vi "ListBox Playground.vi"() -> ()   [LabVIEW 2019]
uses:
  <vilib>/event_ctls.llb/lveventtype.ctl
  <vilib>/event_ctls.llb/eventsource.ctl
  <vilib>/picture/picture.llb/imagedata.ctl
  <vilib>/addons/_JKI Toolkits/Caraya/classes/Test Result/Test Node (Extended).ctl
  <vilib>/addons/_JKI Toolkits/Caraya/classes/Test Result/Test Registration Data.ctl
  <vilib>/Utility/miscctls.llb/LVRowAndColumnUnsignedTypeDef.ctl
  <vilib>/Utility/miscctls.llb/LVRowAndColumnTypeDef.ctl
  <vilib>/addons/_JKI Toolkits/Caraya/classes/Test Result/Test Result.lvclass
panel:
  out "2D Picture 2":picture
  out "image data 2":T1
  out "image data":T1
  out "2D Picture":picture
  out "Ready? 2":bool
  in  "Multicolumn Listbox 2":i32(listbox)
  in  "Patterns":i32(listbox) caption="Patterns (drag-and-drop reorder)"
  out "x = y?":bool
  out "Ctrl":bool
  out "element":string
  out "initialized array":i32[](array[numeric])
  out "Item Names 2":string[][](array[string])
  in  "Multicolumn Listbox":i32(listbox)
  out "Edit Tree Items:Add Item":string
  in  "Tree":string(tree)
  out "Array":string[](array[string])
  out "Item Names":string[](array[string])
  out "Time":u32
  out "Source":T2 items=["LabVIEW UI"=0, "ActiveX"=1, "User Event"=25]
  out "Type":T3=enum."Value Change"
  out "Result":enum16{"Drop Cancel", "Drop Move", "Drop Copy"}(ring)
  out "Drag Ended":bool
  out "Drag Started":bool
  in  "Boolean":bool
  in  "Listbox":i32(listbox)
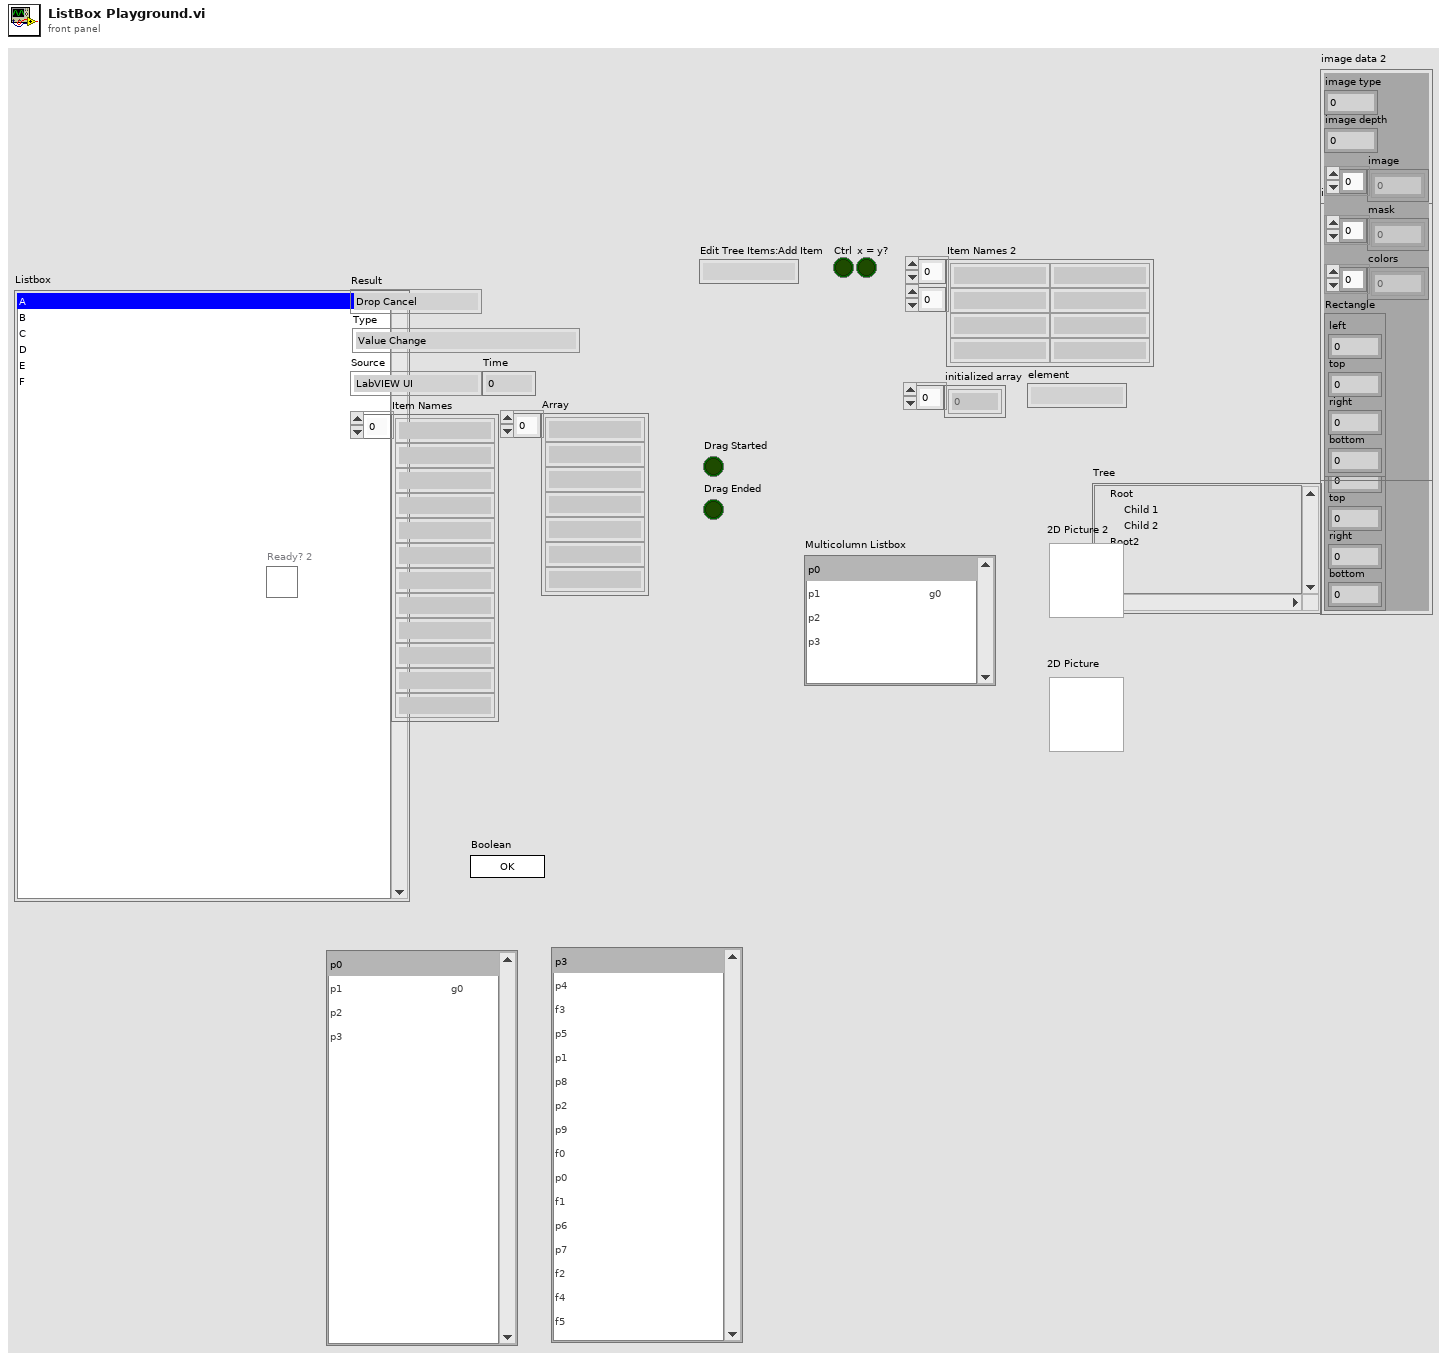
[diagram p1: front panel]
types:
  T1 = typedef "imagedata.ctl" = cluster{"image type":i32, "image depth":i32, "image":u8[], "mask":u8[], "colors":u32[], "Rectangle":cluster{"left":i16, "top":i16, "right":i16, "bottom":i16}}
  T2 = typedef "eventsource.ctl" = u32
  T3 = typedef "lveventtype.ctl" = enum32{"Null", "Timeout", "Annotation Menu Selection", "Annotation Menu Selection?", "App Instance Close", "App Instance Close?", "Autoscale Range Change", "Bookmark Info Change", "Cell Edit", "Cell Edit?", "Cursor Grab", "Cursor Grab?", "Cursor Menu Selection", "Cursor Menu Selection?", "Cursor Move", "Cursor Release", "Data Change", "Direction Change", "Display State Change", "Drag Ended", "Drag Enter", "Drag Leave", "Drag Over", "Drag Source Update", "Drag Starting", "Drag Starting?", "Drop", "Exec State Change", "Key Down", "Key Down?", "Key Repeat", "Key Repeat?", "Key Up", "Listbox Double Click", "Menu Activation?", "Menu Selection (App)", "Menu Selection? (App)", "Menu Selection (User)", "Mouse Down", "Mouse Down?", "Mouse Enter", "Mouse Leave", "Mouse Move", "Mouse Up", "Mouse Wheel", "NI Security User Change (App)", "Pane Size", "Panel Close", "Panel Close?", "Panel Resize", "Plot Attribute Change", "Scale Range Change", "Shortcut Menu Activation?", "Shortcut Menu Selection (App)", "Shortcut Menu Selection? (App)", "Shortcut Menu Selection (User)", "Tree Double Click", "Tree Drag", "Tree Drag?", "Tree Drop", "Tree Drop?", "Tree Item Close", "Tree Item Close?", "Tree Item Open", "Tree Item Open?", "User Event", "Value Change"}
  T4 = cluster{"left":i16, "top":i16, "right":i16, "bottom":i16}
  T5 = typedef "LVRowAndColumnTypeDef.ctl" = cluster{"Row":i32, "Column":i32}
  T6 = typedef "LVRowAndColumnUnsignedTypeDef.ctl" = cluster{"Row":u32, "Column":u32}
  T7 = typedef "Caraya.lvlib/Test Result.lvclass/Test Node (Extended).ctl" = cluster{"Test Registration":T8, "Defined":bool, "Passed":bool, "properties":variant}
  T8 = typedef "Caraya.lvlib/Test Result.lvclass/Test Registration Data.ctl" = cluster{"Name":string, "Call Chain":string[], "Time Stamp":timestamp, "Test ID":string, "Caller ID":string}
  T9 = typedef "LVPoint32TypeDef.ctl" = cluster{"Horizontal":i32, "Vertical":i32}
  T10 = cluster{"Shift":bool, "Ctrl":bool, "Alt":bool, "Cmd":bool, "Opt":bool}
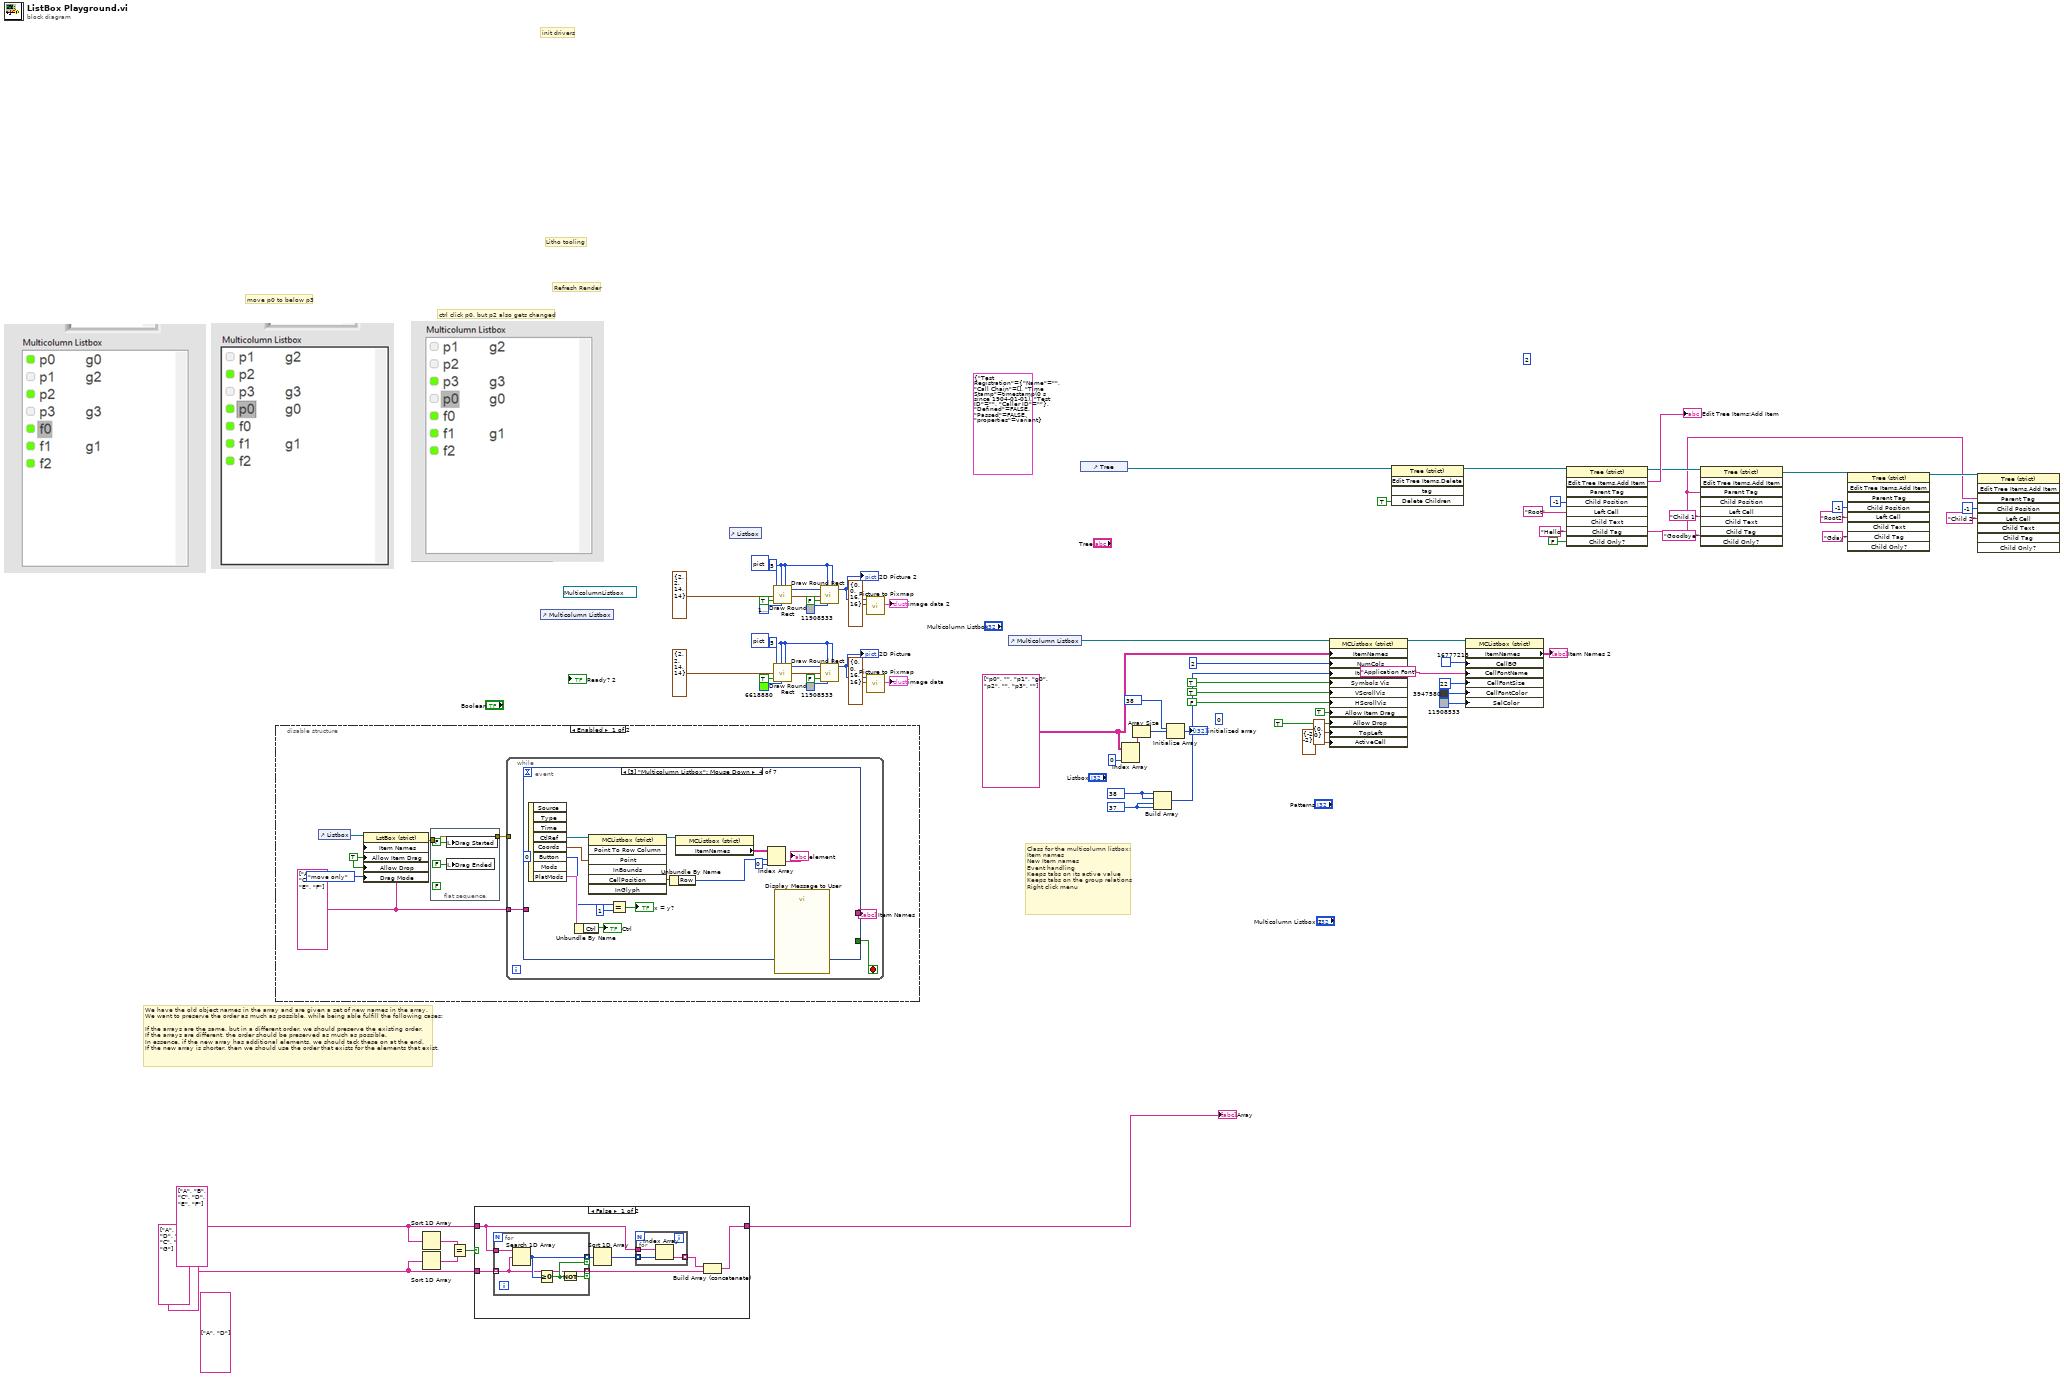
[diagram p0: block diagram]
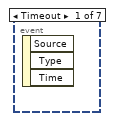
[diagram p3: hidden frame]
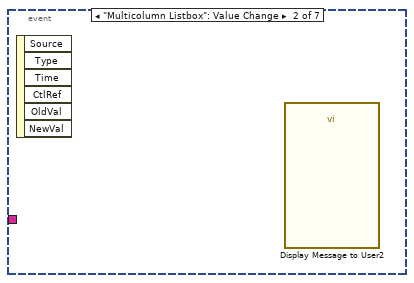
[diagram p4: hidden frame]
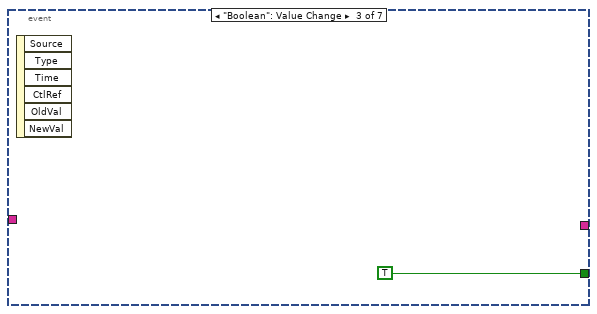
[diagram p5: hidden frame]
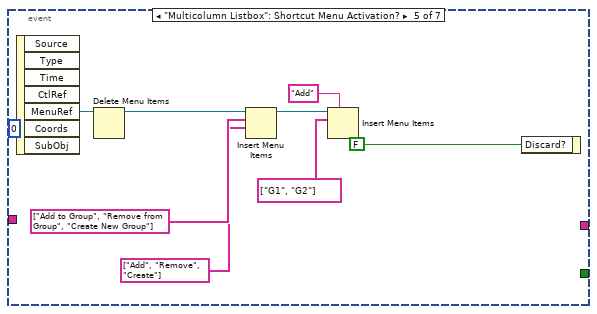
[diagram p6: hidden frame]
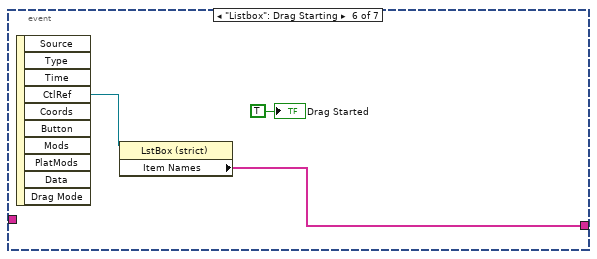
[diagram p7: hidden frame]
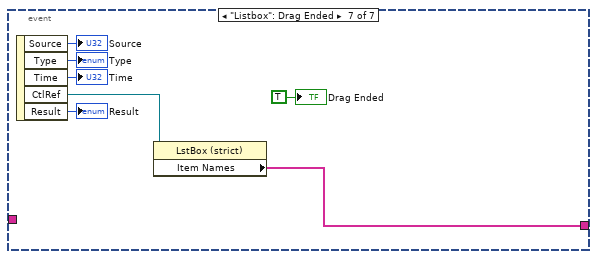
[diagram p8: hidden frame]
diagram:
  w11 = i16 5 ("oval width")
  w7 = T4 {"left"=2, "top"=2, "right"=14, "bottom"=14} ("rect")
  w12 = i16 5 ("oval width")
  w16 = T4 {"left"=2, "top"=2, "right"=14, "bottom"=14} ("rect")
  (unwired) refnum<vi> refnum ("Multicolumn Listbox")
  w36 = 37
  w37 = 38
  (unwired) 0
  w43 = string[][] [["p0", ""], ["p1", "g0"], ["p2", ""], ["p3", ""]] ("Item Names")
  w50 = "Hello" ("Child Tag")
  (unwired) 2
  (unwired) T7 {"Test Registration"={"Name"="", "Call Chain"=[], "Time Stamp"=timestamp(0 s since 1904-01-01), "Test ID"="", "Caller ID"=""}, "Defined"=FALSE, "Passed"=FALSE, "properties"=variant} ("Test Node")
  w67 = string[] ["A", "C", "B", "D", "E", "F"] ("Item Names")
  (unwired) string[] ["A", "D"] ("Item Names")
  (unwired) string[] ["A", "B", "D", "E", "C", "F", "G"] ("Item Names")
  w66 = string[] ["A", "B", "C", "D", "E", "F"] ("Item Names")
  # "ctrl click p0, but p2 also gets changed"
  # "move p0 to below p3"
  # "Class for the multicolumn listbox:\nItem names\nNew Item names\nEvent handling\nKeeps tabs on its active value\nKeeps tabs on the group relations\nRight click menu"
  # "We have the old object names in the array and are given a set of new names in the array.\nWe want to preserve the order as much as possible, while being able fulfill the following cases:\n\nIf the arrays are the same, but in a different order, we should preserve the existing order.\nIf the arrays are different, the order should be preserved as much as possible. \nIn essence, if the new array has additional elements, we should tack these on at the end. \nIf the new array is shorter, then we should use the order that exists for the elements that exist."
  # "Litho tooling"
  # "Refresh Render"
  # "init drivers"
  n1 = disable-structure shown="Enabled" {
    frame Enabled {
      w76 = TRUE ("Drag/Drop:Allow Dragging")
      w75 = string[] ["A", "B", "C", "D", "E", "F"] ("Item Names")
      n2 = control-ref of="Listbox"() -> (w77:refnum<vi>)
      n3 = property class="LstBox (strict)"(reference=w77, "Item Names"=w75, "Allow Item Drag"=w76, "Allow Drop"=w76, "Drag Mode"=enum32{"copy or move", "copy only", "move only"}."move only" ("Drag/Drop:Drag Mode")) -> (error out=w73:errorcluster)  [unwired: 1 in, 1 out]
      n4 = flat-sequence {
        tunnel: [w78] -> w74
        tunnel: w73 -> [w78]
        frame #0 {
          (unwired) FALSE ("Drop")
          n5 = local write "Drag Started"(FALSE ("Drag Started")) -> ()
          n6 = local write "Drag Ended"(FALSE ("Drag Ended")) -> ()
        }
      }
      n7 = while {
        tunnel: w75 -> [w82]
        tunnel: w74 -> [_]
        stop <- w83 stop-if-true
        n8 = event shown="[3] \"Multicolumn Listbox\": Mouse Down" {
          selector: _ -> [_ _ _ _ _ _ _]
          dyn-events: _ -> [_ _ _ _ _ _ _]
          timeout: _ -> [_ _ _ _ _ _ _]
          tunnel: [_ _ TRUE _ _ _ _] -> w83
          tunnel: w82 -> [_ _ _ _ _ _ _]
          tunnel: [_ _ _ _ _ w106 w109] -> w81
          event Timeout {
            n9 = event-data() -> ()  [unwired: 1 in, 3 out]
          }
          event "Multicolumn Listbox": Value Change {
            n10 = event-data() -> ()  [unwired: 1 in, 6 out]
            n11 = call "Display Message to User2"() -> ()  [unwired: 10 in, 2 out]
          }
          event "Boolean": Value Change {
            n12 = event-data() -> ()  [unwired: 1 in, 6 out]
          }
          event "Multicolumn Listbox": Mouse Down {
            (unwired) u16 0 ("Button")
            n13 = event-data() -> ("CtlRef"=w96:refnum<vi>, "Coords"=w95:T9, "Button"=w87:u16, "PlatMods"=w97:T10)  [unwired: 1 in, 4 out]
            n14 = Unbundle By Name(w97) -> ("Ctrl"=→"Ctrl":bool)
            n15 = invoke class="MCListbox (strict)" method="Point To Row Column"(reference=w96, "Point"=w95) -> (reference out=w93:refnum<vi>, "CellPosition"=w94:T5)  [unwired: 5 in, 5 out]
            n16 = Equal?(x=w87, y=u16 1) -> (x = y?=→"x = y?":bool)
            n17 = Unbundle By Name(w94) -> ("Row"=w91:i32)
            n18 = property class="MCListbox (strict)"(reference=w93) -> ("ItemNames"=w92:string[][])  [unwired: 1 in, 2 out]
            n19 = Index Array(array=w92, index (row)=w91, index (col)=0 ("disabled index (col)")) -> (element=→"element":string)
            n20 = call "Display Message to User"() -> ()  [unwired: 10 in, 2 out]
          }
          event "Multicolumn Listbox": Shortcut Menu Activation? {
            (unwired) u16 0 ("Button")
            n21 = event-data() -> ("MenuRef"=w103:refnum<k9>)  [unwired: 1 in, 6 out]
            n22 = Delete Menu Items(9:w103) -> (3:w102:refnum<k9>)  [unwired: 3 in, 1 out]
            n23 = Insert Menu Items(7:string[] ["Add", "Remove", "Create"] ("item tags"), 8:string[] ["Add to Group", "Remove from Group", "Create New Group"] ("item names"), 9:w102) -> (3:w101:refnum<k9>)  [unwired: 3 in, 2 out]
            n24 = Insert Menu Items(5:"Add" ("menu tag"), 8:string[] ["G1", "G2"] ("item names"), 9:w101) -> ()  [unwired: 3 in, 3 out]
            n25 = event-data("Discard?"=FALSE) -> ()  [unwired: 1 in, 1 out]
          }
          event "Listbox": Drag Starting {
            n26 = event-data() -> ("CtlRef"=w107:refnum<vi>)  [unwired: 1 in, 9 out]
            n27 = property class="LstBox (strict)"(reference=w107) -> ("Item Names"=w106:string[])  [unwired: 1 in, 2 out]
            "Drag Started" <- TRUE ("Drag Started")
          }
          event "Listbox": Drag Ended {
            n28 = event-data() -> ("Source"=→"Source":T2, "Type"=→"Type":T3, "Time"=→"Time":u32, "CtlRef"=w110:refnum<vi>, "Result"=→"Result":enum16{"Drop Cancel", "Drop Move", "Drop Copy"})  [unwired: 1 in]
            n29 = property class="LstBox (strict)"(reference=w110) -> ("Item Names"=w109:string[])  [unwired: 1 in, 2 out]
            "Drag Ended" <- TRUE ("Drag Ended")
          }
        }
        "Item Names" <- w81
      }
    }
    frame Disabled {
    }
  }
  n30 = Sort 1D Array(array=w66) -> (sorted array=w71:string[])
  n31 = Sort 1D Array(array=w67) -> (sorted array=w70:string[])
  n32 = Equal?(x=w71, y=w70) -> (x = y?=w69:bool)
  n33 = case shown="False" w69 {
    tunnel: w66 -> [w116 w131]
    tunnel: w67 -> [w120 _]
    tunnel: [w121 w131] -> w68
    frame False {
      n34 = for {
        tunnel: w116 -> [w129]
        tunnel: w120 -> [w126] mode=indexing
        tunnel: [w126] -> w122 mode=indexing if=w130
        tunnel: [w128] -> w119 mode=indexing if=w127
        n35 = Search 1D Array(1D array=w129, element=w126) -> (index of element=w128:i32)  [unwired: 1 in]
        n36 = Greater Or Equal To 0?(x=w128) -> (x >= 0?=w127:bool)
        n37 = Not(x=w127) -> (.not. x?=w130:bool)
      }
      n38 = Sort 1D Array(array=w119) -> (sorted array=w118:i32[])
      n39 = for {
        tunnel: w116 -> [w125]
        tunnel: w118 -> [w124] mode=indexing
        tunnel: [w123] -> w117 mode=indexing
        n40 = Index Array(array=w125, index=w124) -> (element=w123:string)
      }
      n41 = Build Array (concatenate)(w117, w122) -> (w121:string[])
    }
    frame True {
    }
  }
  "Array" <- w68
  n42 = control-ref of="Multicolumn Listbox"() -> ()  [unwired: 1 out]
  n43 = control-ref of="Listbox"() -> ()  [unwired: 1 out]
  n44 = call <vilib>:"Draw Round Rect.vi"("picture"=picture data[5B], "oval width"=w11, "rect"=w7, "fill?(F)"=TRUE, "color(black)"=u32 16777238, "oval height"=w11) -> ("new picture"=w6:picture)  [unwired: 3 in]
  n45 = call <vilib>:"Draw Round Rect.vi"("picture"=picture data[5B], "oval width"=w12, "rect"=w16, "fill?(F)"=TRUE, "color(black)"=u32 6618880, "oval height"=w12) -> ("new picture"=w17:picture)  [unwired: 3 in]
  n46 = call <vilib>:"Draw Round Rect.vi"("picture"=w6, "oval width"=w11, "rect"=w7, "fill?(F)"=FALSE, "color(black)"=u32 11908533, "oval height"=w11) -> ("new picture"=w8:picture)  [unwired: 3 in]
  "2D Picture 2" <- w8
  n47 = call <vilib>:"Draw Round Rect.vi"("picture"=w17, "oval width"=w12, "rect"=w16, "fill?(F)"=FALSE, "color(black)"=u32 11908533, "oval height"=w12) -> ("new picture"=w15:picture)  [unwired: 3 in]
  "2D Picture" <- w15
  n48 = call <vilib>:"Picture to Pixmap.vi"("rect"=T4 {"left"=0, "top"=0, "right"=16, "bottom"=16}, "picture"=w8) -> ("image data"=→"image data 2":T1)  [unwired: 8 in, 1 out]
  n49 = call <vilib>:"Picture to Pixmap.vi"("rect"=T4 {"left"=0, "top"=0, "right"=16, "bottom"=16}, "picture"=w15) -> ("image data"=→"image data":T1)  [unwired: 8 in, 1 out]
  n50 = control-ref of="Multicolumn Listbox"() -> (w46:refnum<vi>)
  n51 = control-ref of="Tree"() -> (w64:refnum<vi>)
  n52 = Index Array(array=w43, index (col)=0 ("disabled index (col)")) -> (element=w41:string[])  [unwired: 1 in]
  n53 = Array Size(array=w41) -> (size(s)=w40:i32)
  n54 = Build Array(w37, w37, w36, w36) -> (w35:i32[])
  n55 = Initialize Array(38, w40) -> (→"initialized array":i32[])
  n56 = property class="MCListbox (strict)"(reference=w46, "ItemNames"=w43, "NumCols"=u32 2 ("Number of Columns"), "ItemSyms"=w35, "Symbols Vis"=TRUE ("Visible Items:Symbols Visible"), "VScrollVis"=TRUE ("Visible Items:Vertical Scrollbar Visible"), "HScrollVis"=FALSE ("Visible Items:Horizontal Scrollbar Visible"), "Allow Item Drag"=TRUE ("Drag/Drop:Allow Dragging"), "Allow Drop"=TRUE ("Drag/Drop:Allow Dropping"), "TopLeft"=T6 {"Row"=0, "Column"=0} ("Top Left Visible Cell"), "ActiveCell"=T5 {"Row"=-2, "Column"=-2} ("Active Cell:Active Cell")) -> (reference out=w34:refnum<vi>)  [unwired: 1 in, 1 out]
  n57 = invoke class="Tree (strict)" method="Edit Tree Items.Delete"(reference=w64, "Delete Children"=TRUE ("Delete Children?")) -> (reference out=w62:refnum<vi>)  [unwired: 3 in, 4 out]
  n58 = property class="MCListbox (strict)"(reference=w34, "CellBG"=u32 16777215 ("Active Row:Cell Background Color"), "CellFontName"="Application Font" ("Font Name"), "CellFontSize"=u32 22 ("Size"), "CellFontColor"=u32 3947580 ("Color"), "SelColor"=u32 11908533 ("Active Row:Cell Background Color")) -> ("ItemNames"=→"Item Names 2":string[][])  [unwired: 1 in, 2 out]
  n59 = invoke on="Invoke Node" class="Tree (strict)" method="Edit Tree Items.Add Item"(reference=w62, "Child Position"=-1, "Left Cell"="Root" ("Name"), "Child Tag"=w50, "Child Only?"=FALSE) -> (reference out=w58:refnum<vi>, "Edit Tree Items:Add Item"=→"Edit Tree Items:Add Item":string)  [unwired: 4 in, 7 out]
  n60 = invoke on="Invoke Node" class="Tree (strict)" method="Edit Tree Items.Add Item"(reference=w58, "Parent Tag"=w50, "Left Cell"="Child 1" ("Left Cell String"), "Child Tag"="Goodbye") -> (reference out=w55:refnum<vi>)  [unwired: 5 in, 8 out]
  n61 = invoke on="Invoke Node" class="Tree (strict)" method="Edit Tree Items.Add Item"(reference=w55, "Child Position"=-1, "Left Cell"="Root2" ("Left Cell String"), "Child Tag"="Gday") -> (reference out=w51:refnum<vi>)  [unwired: 5 in, 8 out]
  n62 = invoke on="Invoke Node" class="Tree (strict)" method="Edit Tree Items.Add Item"(reference=w51, "Parent Tag"=w50, "Child Position"=-1, "Left Cell"="Child 2" ("Left Cell String")) -> ()  [unwired: 5 in, 9 out]
